vi "Initialize.vi"(8 "error in (no error)":errorcluster, 11 "DemoMicrosope in":refnum<class "DemoMicrosope.lvclass">) -> (0 "error out":errorcluster, 3 "DemoMicrosope out":refnum<class "DemoMicrosope.lvclass">)   [LabVIEW 2020]
uses:
  <vilib>/ActorFramework/Actor/Actor.lvclass
  DemoStage/DemoStage/DemoStage.lvclass
  C:/Program Files/National Instruments/LabVIEW 2020/vi.lib/ActorFramework/Actor/Actor.lvclass
  DemoMicrosope.lvclass
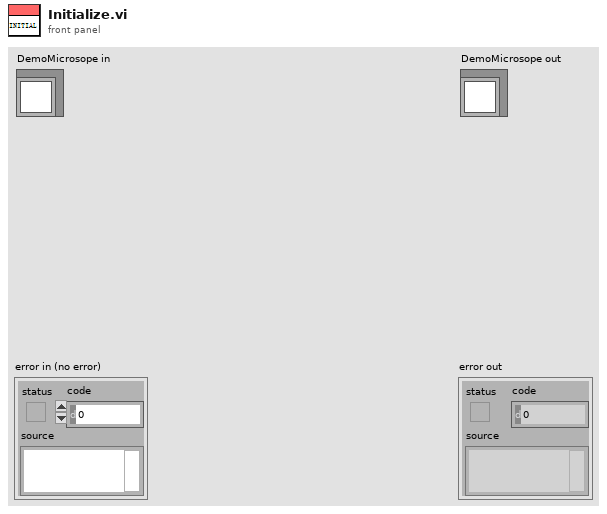
[diagram p1: front panel]
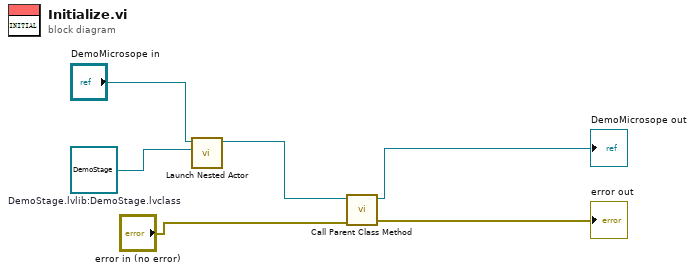
[diagram p0: block diagram]
diagram:
  w1 = refnum<class "DemoStage.lvclass"> refnum  # DemoStage.lvlib:DemoStage.lvclass
  n1 = call <vilib>:"Launch Nested Actor.vi"("Nested Actor"=w1, "Caller Actor in"="DemoMicrosope in") -> ("Caller Actor out"=w2:refnum<class "DemoMicrosope.lvclass">)  [unwired: 7 in, 2 out]
  n2 = call-parent "Call Parent Class Method"("error in (no error)"="error in (no error)", "Microscope in"=w2) -> ("error out"=→"error out":errorcluster, "Microscope out"=→"DemoMicrosope out":refnum<class "DemoMicrosope.lvclass">)  [unwired: 8 in]
